vi "LINC Get Definition File Paths.vi"(8 "error in (no error)":errorcluster, 11 "LINC session":refnum<class "LINC.lvclass">) -> (0 "error out":errorcluster, 1 "TLM defintion path":path, 2 "CMD definition path":path, 3 "dup LINC session":refnum<class "LINC.lvclass">, 5 "CMD definition exists":bool, 7 "TLM definition exists":bool)   [LabVIEW 2018, in "STEPkgDriver_LINC.lvlib" / "LINC.lvclass"]
uses:
  LINC.lvclass
  STEPkgDriver_LINC.lvlib
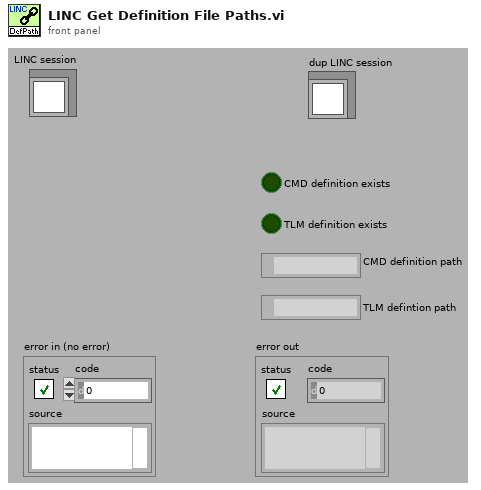
[diagram p1: front panel]
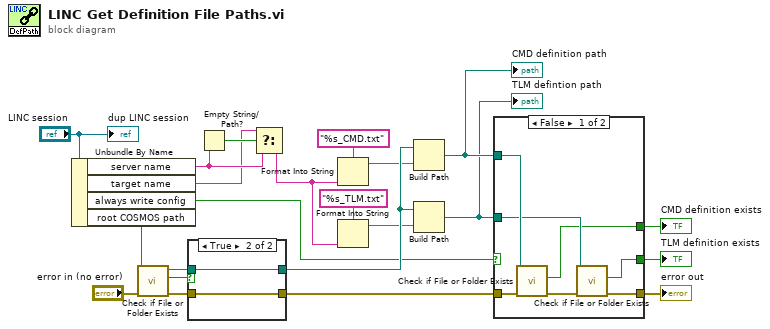
[diagram p0: block diagram]
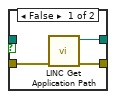
[diagram p2: hidden frame]
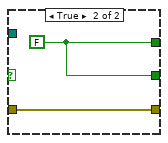
[diagram p3: hidden frame]
diagram:
  n1 = Unbundle By Name("LINC session") -> ("server name"=w6:string, "target name"=w5:string, "always write config"=w2:bool, "root COSMOS path"=w1:path)
  n2 = call <vilib>:"Check if File or Folder Exists.vi"("error in (no error)"="error in (no error)", "path"=w1) -> ("error out"=w11:errorcluster, "file or folder exists?"=w10:bool, "dup path"=w9:path)  [unwired: 7 in]
  n3 = case shown="True" w10 {
    tunnel: [w23 w26] -> w22
    tunnel: w11 -> [w25 w27]
    tunnel: [w24 w27] -> w17
    tunnel: w9 -> [_ w26]
    frame False {
      n4 = call "LINC Get Application Path.vi"("error in (no error)"=w25) -> ("error out"=w24:errorcluster, "application path"=w23:path)  [unwired: 9 in]
    }
    frame True {
    }
  }
  n5 = Empty String/Path?(string/path=w6) -> (empty?=w7:bool)
  n6 = Select(t=w5, s=w7, f=w6) -> (s? t:f=w4:string)
  n7 = Format Into String(format string="%s_CMD.txt", w4) -> (resulting string=w18:string)  [unwired: 2 in, 1 out]
  n8 = Format Into String(format string="%s_TLM.txt", w4) -> (resulting string=w20:string)  [unwired: 2 in, 1 out]
  n9 = Build Path(base path=w22, name or relative path=w18) -> (appended path=w16:path)
  "CMD definition path" <- w16
  n10 = Build Path(base path=w22, name or relative path=w20) -> (appended path=w14:path)
  "TLM defintion path" <- w14
  n11 = case shown="False" w2 {
    tunnel: w17 -> [w34 w35]
    tunnel: w16 -> [w33 _]
    tunnel: [w31 w35] -> w15
    tunnel: w14 -> [w30 _]
    tunnel: [w29 w36] -> w13
    tunnel: [w28 w36] -> w12
    frame False {
      n12 = call <vilib>:"Check if File or Folder Exists.vi"("error in (no error)"=w34, "path"=w33) -> ("error out"=w32:errorcluster, "file or folder exists?"=w29:bool)  [unwired: 7 in, 1 out]
      n13 = call <vilib>:"Check if File or Folder Exists.vi"("error in (no error)"=w32, "path"=w30) -> ("error out"=w31:errorcluster, "file or folder exists?"=w28:bool)  [unwired: 7 in, 1 out]
    }
    frame True {
      w36 = FALSE ("file or folder exists?")
    }
  }
  "error out" <- w15
  "CMD definition exists" <- w13
  "TLM definition exists" <- w12
  "dup LINC session" <- "LINC session"
